vi "Global FieldWidthY.vi"() -> ()   [LabVIEW 2014]
panel:
  out "FieldWidthY":dbl=50.0
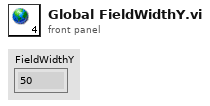
[diagram p1: front panel]
diagram:
